vi "third childs(json).vi"(6 "pointSpec":string[][](array[string]), 7 "StatusRef":refnum<vi>, 8 "SN":string, 9 "third test item name":string, 10 "third result":string[][](array[string]), 11 "all rows":string[][](array[string]) caption="dataSource") -> (0 "thirdChilds":string)   [LabVIEW 2011]
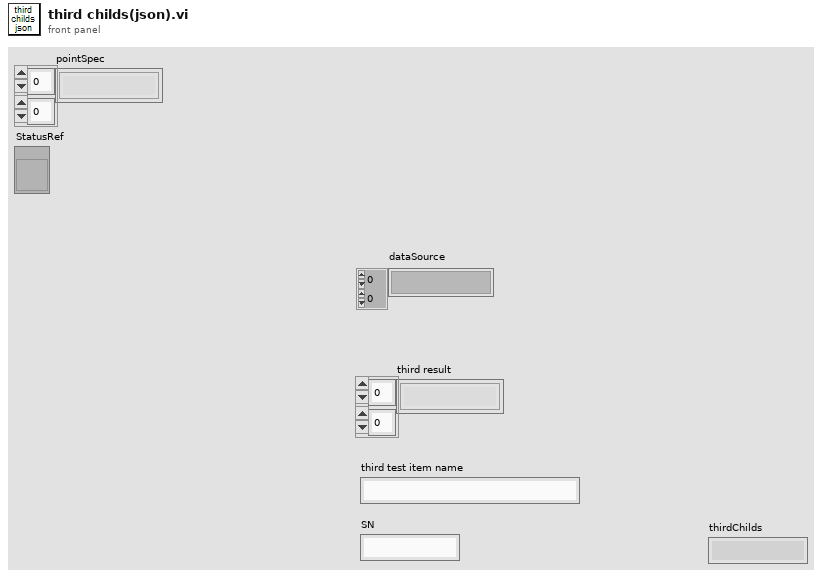
[diagram p1: front panel]
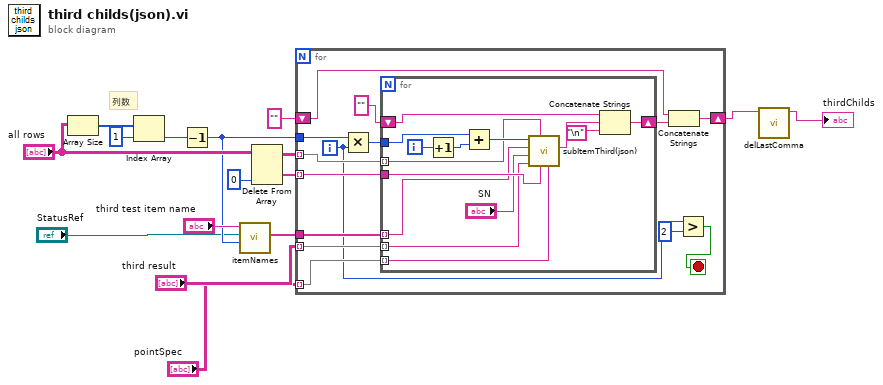
[diagram p0: block diagram]
diagram:
  # "列数"
  n1 = Array Size(array="all rows") -> (size(s)=w16:i32[])
  n2 = Index Array(array=w16, index=1 ("索引")) -> (element=w8:i32)
  n3 = Decrement(x=w8) -> (x-1=w6:i32)
  n4 = call "itemNames.vi"("pair"=w6, "StatusRef"="StatusRef", "itemName"="third test item name") -> ("itemNameArray"=w7:string[])  [unwired: 8 in]
  n5 = Delete From Array(array="all rows", index (col)=0 ("禁用的索引 (列)")) -> (deleted portion=w10:string[], array with subset deleted=w11:string[][])  [unwired: 2 in]
  n6 = for {
    tunnel: w6 -> [w30]
    tunnel: "third result" -> [w28] mode=indexing
    shift-right: [w24] -> w3
    shift-left: "" -> [w26]
    tunnel: w11 -> [w23] mode=indexing
    tunnel: w10 -> [w22] mode=indexing
    tunnel: w7 -> [w21]
    tunnel: "pointSpec" -> [w20] mode=indexing
    i -> [w19]
    stop <- w17 stop-if-true
    n7 = Multiply(x=w30, y=w19) -> (x*y=w29:i32)
    n8 = for {
      tunnel: w23 -> [w41] mode=indexing
      tunnel: w29 -> [w44]
      tunnel: w22 -> [w42]
      tunnel: w28 -> [w40] mode=indexing
      shift-right: [w35] -> w25
      shift-left: "" -> [w37]
      tunnel: w21 -> [w32] mode=indexing
      tunnel: w20 -> [w31] mode=indexing
      i -> [w34]
      n9 = Increment(x=w34) -> (x+1=w33:i32)
      n10 = Add(x=w44, y=w33) -> (x+y=w43:i32)
      n11 = call "subItemThird(json).vi"("pointLimit"=w31, "single frequency"=w42, "single frequency value"=w41, "single frequency result"=w40, "SN"="SN", "third test item name"=w32, "subIDcount"=w43) -> ("SubItem"=w36:string)  [unwired: 4 in]
      n12 = Concatenate Strings(w37, w36, "\n") -> (w35:string)
    }
    n13 = Concatenate Strings(w26, w25) -> (w24:string)
    n14 = Greater?(x=w19, y=2) -> (0:w17:bool)
  }
  n15 = call "delLastComma.vi"("字符串"=w3) -> ("result string"=→"thirdChilds":string)  [unwired: 10 in]
